vi "Configure AI Module.vi"(0 "VISA resource name":refnum<visa-resource-name>, 1 "A/D Integrate (0: Auto)":u16(ring) items=["Auto", "50Hz", "60Hz", "Common"], 2 "Burnout Set":T1={"Change Burnout Set (False)"=FALSE, "Lower Limit (-10.0)"=-10.0, "Upper Limit (110.0)"=110.0} {"Upper Limit (110.0)" min=105.0 max=120.0 step=0.1 format="%.1f"; "Lower Limit (-10.0)" min=-20.0 max=-5.0 step=0.1 format="%.1g"}, 5 "Unit Number (0)":i32 min=0 max=6 step=1, 7 "Module Number (0)":i32 min=0 max=9 step=1, 9 "Operation Mode (1: 10CH)":u16(ring)=1 items=["2CH", "10CH", "6CH", "4CH"], 11 "error in (no error)":errorcluster, 12 "Module Kind (0: AI)":u16(ring) items=["AI", "AI (mA)"]) -> (4 "VISA resource name out":refnum<visa-resource-name>, 6 "Unit Number":i32, 8 "Module Number":i32, 15 "error out":errorcluster)   [LabVIEW 2020, in "Yokogawa GX Series.lvlib"]
doc: "Sets the mode and A/D integration time of an AI module.\n\nThe combinations of mode and A/D integral time vary depending on the interval time. See the instrument communication command User's Manual.\n\nCommand: SModeAI"
uses:
  <instrlib>/Yokogawa GX Series/Yokogawa GX Series.lvlib
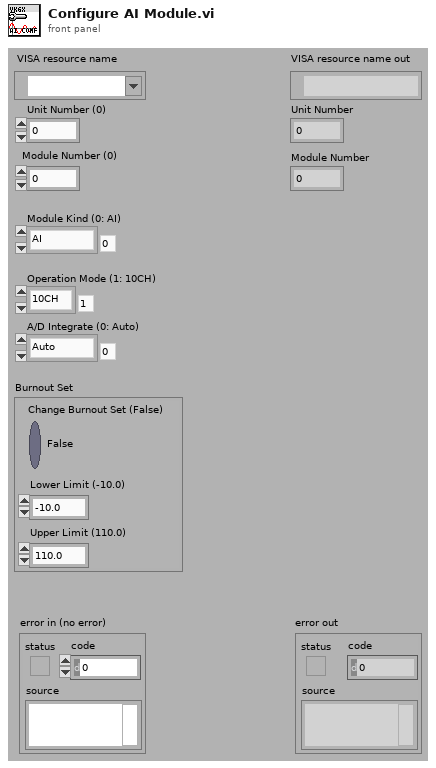
[diagram p1: front panel]
types:
  T1 = cluster{"Change Burnout Set (False)":bool, "Lower Limit (-10.0)":dbl, "Upper Limit (110.0)":dbl}
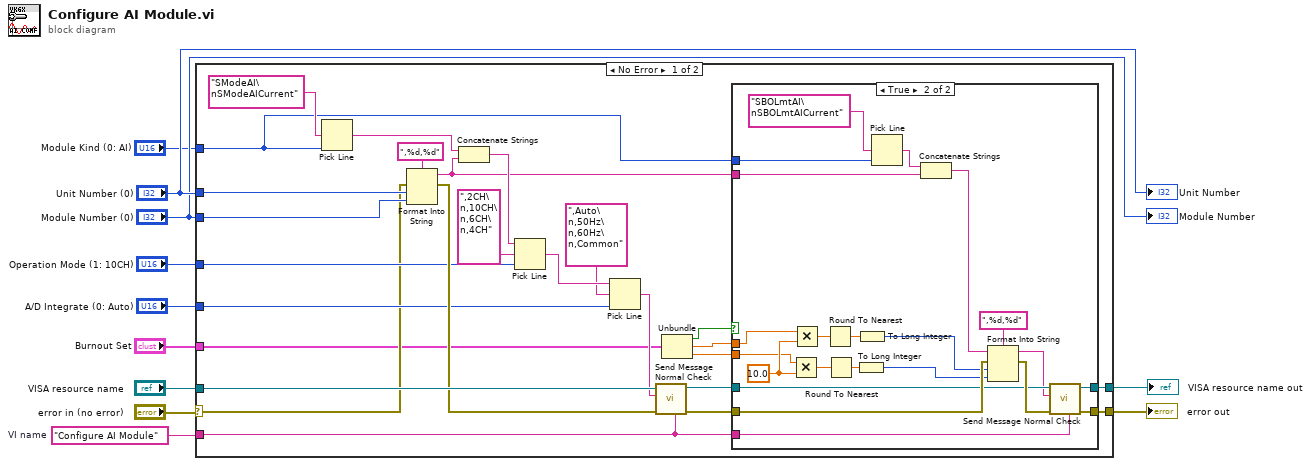
[diagram p0: block diagram]
diagram:
  w3 = "Configure AI Module"  # VI name
  n1 = case shown="No Error" "error in (no error)" {
    selector: "error in (no error)" -> [w26 w62]
    tunnel: "VISA resource name" -> [w36 w63]
    tunnel: [w20 w63] -> w10
    tunnel: [w19 w62] -> w9
    tunnel: "Operation Mode (1: 10CH)" -> [w34 _]
    tunnel: "A/D Integrate (0: Auto)" -> [w31 _]
    tunnel: "Unit Number (0)" -> [w28 _]
    tunnel: "Module Number (0)" -> [w27 _]
    tunnel: w3 -> [w12 _]
    tunnel: "Module Kind (0: AI)" -> [w16 _]
    tunnel: "Burnout Set" -> [w23 _]
    frame No Error {
      n2 = Pick Line(multi-line string="SModeAI\nSModeAICurrent", line index=w16) -> (output string=w15:string)  [unwired: 1 in]
      n3 = Format Into String(format string=",%d,%d", error in=w26, w28, w27) -> (resulting string=w13:string, error out=w35:errorcluster)  [unwired: 1 in]
      n4 = Concatenate Strings(w15, w13) -> (w14:string)
      n5 = Pick Line(string ("")=w14, multi-line string=",2CH\n,10CH\n,6CH\n,4CH", line index=w34) -> (output string=w32:string)
      n6 = Pick Line(string ("")=w32, multi-line string=",Auto\n,50Hz\n,60Hz\n,Common", line index=w31) -> (output string=w30:string)
      n7 = call <instrlib>:"Send Message Normal Check.vi"("Source (\"\")"=w12, "error in (no error)"=w35, "Send Message (\"\")"=w30, "VISA resource name"=w36) -> ("error out"=w21:errorcluster, "VISA resource name out"=w22:refnum<visa-resource-name>)  [unwired: 2 in, 4 out]
      n8 = Unbundle(w23) -> ("Change Burnout Set (False)"=w24:bool, "Lower Limit (-10.0)"=w18:dbl, "Upper Limit (110.0)"=w17:dbl)
      n9 = case shown="True" w24 {
        tunnel: w22 -> [w39 w53]
        tunnel: w21 -> [w38 w55]
        tunnel: [w39 w52] -> w20
        tunnel: [w38 w51] -> w19
        tunnel: w18 -> [_ w47]
        tunnel: w17 -> [_ w46]
        tunnel: w16 -> [_ w61]
        tunnel: w13 -> [_ w60]
        tunnel: w12 -> [_ w49]
        frame False {
        }
        frame True {
          w48 = 10.0
          n10 = Multiply(x=w46, y=w48) -> (x*y=w44:dbl)
          n11 = Multiply(x=w47, y=w48) -> (x*y=w45:dbl)
          n12 = Round To Nearest(number=w45) -> (nearest integer value=w43:dbl)
          n13 = Round To Nearest(number=w44) -> (nearest integer value=w42:dbl)
          n14 = To Long Integer(number=w42) -> (32bit integer=w40:i32)
          n15 = To Long Integer(number=w43) -> (32bit integer=w41:i32)
          n16 = Pick Line(multi-line string="SBOLmtAI\nSBOLmtAICurrent", line index=w61) -> (output string=w59:string)  [unwired: 1 in]
          n17 = Concatenate Strings(w59, w60) -> (w57:string)
          n18 = Format Into String(format string=",%d,%d", initial string=w57, error in=w55, w41, w40) -> (resulting string=w50:string, error out=w54:errorcluster)
          n19 = call <instrlib>:"Send Message Normal Check.vi"("Source (\"\")"=w49, "error in (no error)"=w54, "Send Message (\"\")"=w50, "VISA resource name"=w53) -> ("error out"=w51:errorcluster, "VISA resource name out"=w52:refnum<visa-resource-name>)  [unwired: 2 in, 4 out]
        }
      }
    }
    frame Error {
    }
  }
  "error out" <- w9
  "VISA resource name out" <- w10
  "Unit Number" <- "Unit Number (0)"
  "Module Number" <- "Module Number (0)"
